vi "Write LM Read Rate (No Objects).vi"(8 "error in (no error)":errorcluster, 10 "Fast?":bool, 11 "Cluster In":T3={"helium"={"fastHe?"=FALSE, "slowHe?"=FALSE, "fillHe?"=FALSE, "lowHe?"=FALSE}, "nitrogen"={"fillN?"=FALSE, "lowN?"=FALSE}, "Shutdown"=FALSE, "Cryogen Levels"=[], "IO Info"={"Address"={"Com Port"=1, "ISOBUS Address"=5, "GPIB Address"=24, "Communication"=enum."ISOBUS"}, "ILM Name"="", "Display Channel"=[]}} {"Cryogen Levels" min=-1.0 max=100.0 scale=0.0..100.0}) -> (0 "error out":errorcluster, 3 "Cluster Out":T3={"helium"={"fastHe?"=FALSE, "slowHe?"=FALSE, "fillHe?"=FALSE, "lowHe?"=FALSE}, "nitrogen"={"fillN?"=FALSE, "lowN?"=FALSE}, "Shutdown"=FALSE, "Cryogen Levels"=[], "IO Info"={"Address"={"Com Port"=1, "ISOBUS Address"=5, "GPIB Address"=24, "Communication"=enum."ISOBUS"}, "ILM Name"="", "Display Channel"=[]}} {"Cryogen Levels" min=-1.0 max=100.0 scale=0.0..100.0})   [LabVIEW 2012]
uses:
  Cryogen Levels.ctl
  Oxford/BUSGEN.LLB/OxfordAddress.ctl
  Level Meter.lvclass
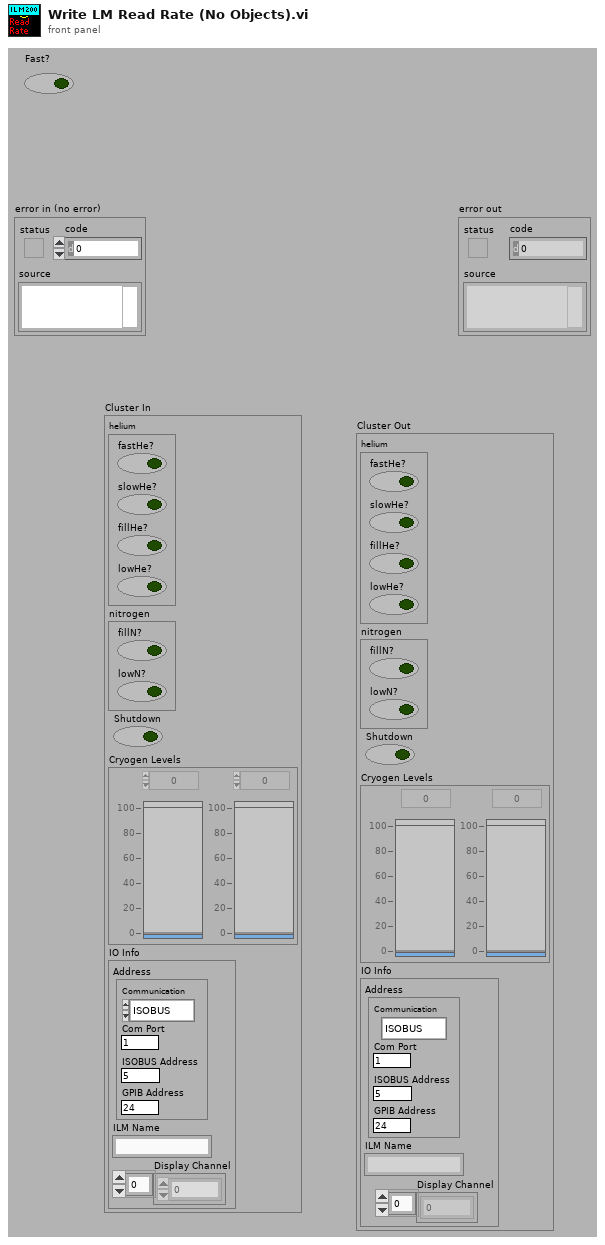
[diagram p1: front panel]
types:
  T1 = typedef "Level Meter.lvclass/Cryogen Levels.ctl" = dbl[]
  T2 = typedef "OxfordAddress.ctl" = cluster{"Com Port":i32, "ISOBUS Address":i32, "GPIB Address":i16, "Communication":enum16{"RS232", "ISOBUS", "GPIB", "Gateway"}}
  T3 = cluster{"helium":cluster{"fastHe?":bool, "slowHe?":bool, "fillHe?":bool, "lowHe?":bool}, "nitrogen":cluster{"fillN?":bool, "lowN?":bool}, "Shutdown":bool, "Cryogen Levels":T1, "IO Info":cluster{"Address":T2, "ILM Name":string, "Display Channel":i32[]}}
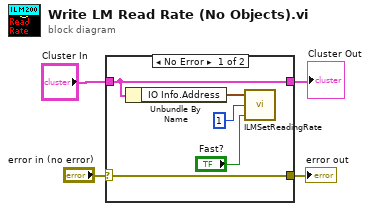
[diagram p0: block diagram]
diagram:
  n1 = case shown="No Error" "error in (no error)" {
    selector: "error in (no error)" -> [w6 w10]
    tunnel: [w6 w10] -> w3
    tunnel: "Cluster In" -> [w5 w11]
    tunnel: [w5 w11] -> w1
    frame No Error {
      n2 = Unbundle By Name(w5) -> ("IO Info.Address"=w8:T2)
      n3 = call "ILMSetReadingRate.vi"("Fast"="Fast?", "Channel(1-3)"=1, "Address"=w8) -> ()  [unwired: 1 out]
    }
    frame Error {
    }
  }
  "error out" <- w3
  "Cluster Out" <- w1
